vi "hybrid_convolution_filter.vi"(11 "input":dbl) -> (3 "output":dbl)   [LabVIEW 2020]
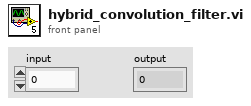
[diagram p1: front panel]
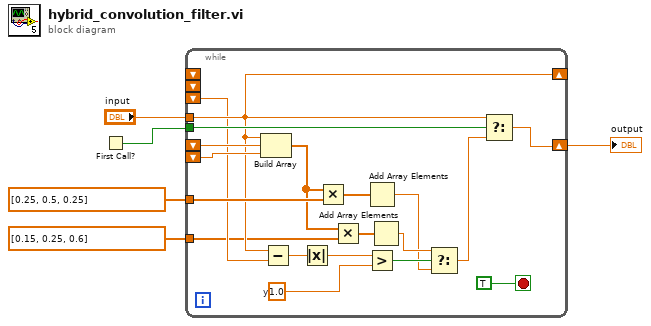
[diagram p0: block diagram]
diagram:
  n1 = First Call?() -> (First Call?: T/F=w2:bool)
  n2 = while {
    tunnel: w2 -> [w23]
    shift-right: [w22] -> w3
    shift-left: _ -> [w21]
    tunnel: "input" -> [w14]
    shift-left: _ -> [w19]
    tunnel: dbl[] [0.25, 0.5, 0.25] -> [w20]
    shift-right: [w14] -> _
    shift-left: _ -> [_]
    shift-left: _ -> [_]
    shift-left: _ -> [w13]
    tunnel: dbl[] [0.15, 0.25, 0.6] -> [w11]
    stop <- TRUE stop-if-true
    w16 = 1.0  # y
    n3 = Build Array(w14, w21, w19) -> (w10:dbl[])
    n4 = Subtract(x=w14, y=w13) -> (x-y=w18:dbl)
    n5 = Absolute Value(x=w18) -> (abs(x)=w17:dbl)
    n6 = Multiply(x=w10, y=w20) -> (x*y=w12:dbl[])
    n7 = Multiply(x=w10, y=w11) -> (x*y=w9:dbl[])
    n8 = Add Array Elements(numeric array=w12) -> (sum=w7:dbl)
    n9 = Greater?(x=w17, y=w16) -> (0:w15:bool)
    n10 = Add Array Elements(numeric array=w9) -> (sum=w8:dbl)
    n11 = Select(t=w8, s=w15, f=w7) -> (s? t:f=w6:dbl)
    n12 = Select(t=w14, s=w23, f=w6) -> (s? t:f=w22:dbl)
  }
  "output" <- w3
